vi "clear_and_initialize_fifos.vi"   [LabVIEW 2015]
uses:
  <vilib>/rvi/Emulation/niFpgaGetClockAttributes.vi
  <vilib>/rvi/Emulation/niFpgaSctlEmulationGetInTimedLoop.vi
  <vilib>/rvi/Emulation/niFpgaEmulationReportErrorSimple.vi
  <vilib>/rvi/Emulation/niFpgaEmulationIsFPGAContextNoSignature.vi
  <vilib>/rvi/FIFO/Fifo_Resource/nirvififoEmulationSetSize.vi
  <vilib>/rvi/DataTransferAndStorage/Container/Common/niFpgaContainerGetUniqueNameForEmu.vi
  <vilib>/rvi/FIFO/Fifo_Resource/nirviFifoEmulationQueueMgr.vi
  <instcachedir>/0/nirviFifoEmulationQueueMgr_E5CAEC123FF24DC58D834DCA3CDAA9B5.lvgen/nirviFifoEmulationQueueMgr_E5CAEC123FF24DC58D834DCA3CDAA9B5_002.vi
  <vilib>/rvi/Emulation/niFpgaProcessEmulError.vi
  <vilib>/rvi/DataTransferAndStorage/Container/Common/niFpgaContainerExecOnDevCompGetState.vi
  <vilib>/rvi/errors/niFpgaSetErrorForExecOnDevCompSimple.vi
  <vilib>/rvi/eio/common/nirviEmuReportErrorAndStop.vi
  <vilib>/rvi/FIFO/Fifo_Resource/nirvififoEmulationDetermineInputValidOut.vi
  <vilib>/rvi/FIFO/Fifo_Resource/nirvififoEmulationCreateLock.vi
  <vilib>/rvi/FIFO/Fifo_Resource/nirvififoEmulationObtainLock.vi
  <vilib>/rvi/FIFO/Fifo_Resource/nirvififoEmulationReleaseLock.vi
  <vilib>/rvi/occurrence/nirviWaitOnOccurrenceBase.vi
  <vilib>/rvi/errors/nirviReportUnexpectedCaseInternalError.vi
  <vilib>/rvi/errors/nirviReportUnexpectedCaseInternalError (U32).vi
  <vilib>/Utility/error.llb/Clear Errors.vi
  <vilib>/rvi/interface/RandomDataEmulation/niFpgaRandomDataHandleErrors.vi
  <vilib>/rvi/Emulation/niFpgaCriticalErrorInLSC.vi
  <instcachedir>/0/nirviFifoEmulationQueueMgr_E5CAEC123FF24DC58D834DCA3CDAA9B5.lvgen/nirviFifoEmulationQueueMgr_E5CAEC123FF24DC58D834DCA3CDAA9B5_001.vi
  <instcachedir>/0/nirviFifoEmulationQueueMgr_E5CAEC123FF24DC58D834DCA3CDAA9B5.lvgen/nirviFifoEmulationQueueMgr_E5CAEC123FF24DC58D834DCA3CDAA9B5_003.vi
  <vilib>/rvi/DataTransferAndStorage/Container/XNode/niFpgaContainer.xnode
  <vilib>/rvi/FIFO/Fifo_Resource/nirvififoEmulationClear.vi
  <vilib>/rvi/FIFO/Fifo_Resource/niFpgaFifoEmulationRefIn.vi
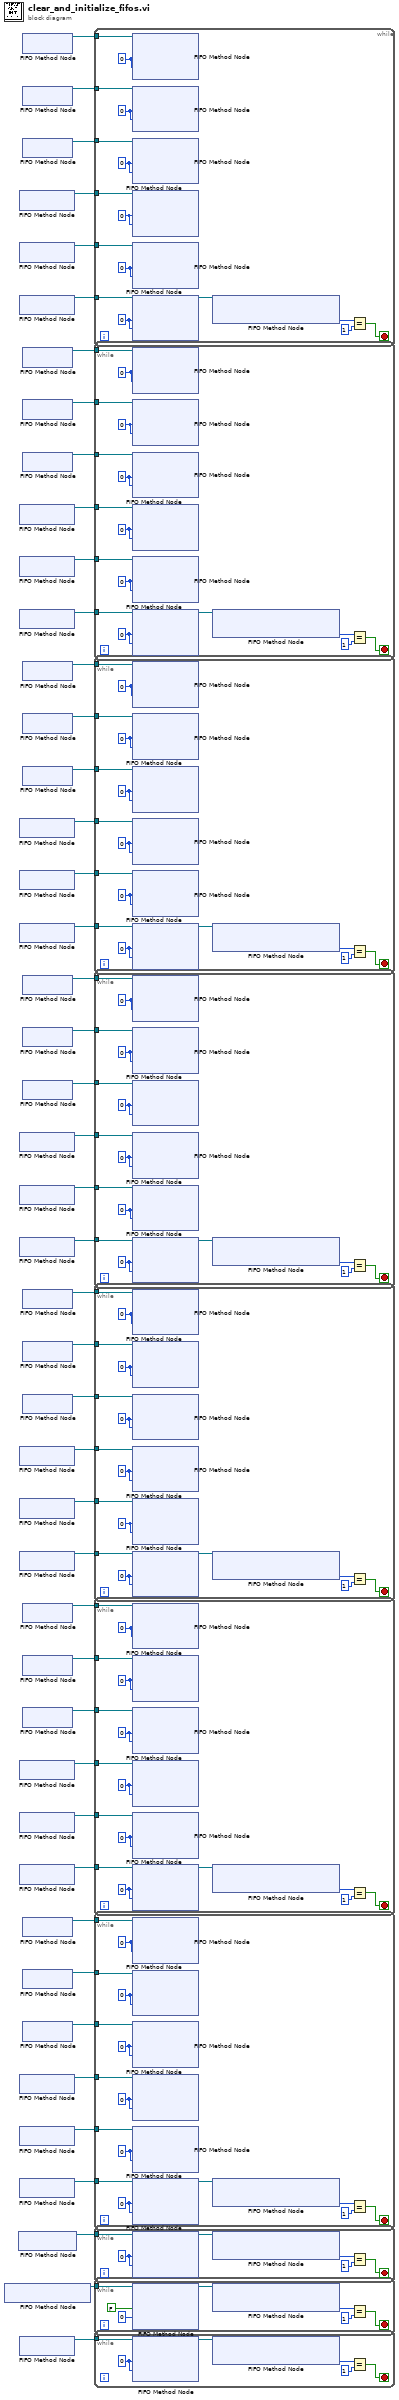
[diagram p0: block diagram]
diagram:
  n1 = xnode ("FIFO Method Node")() -> ("FIFO Out"=w2:refnum<k21>)  [unwired: 1 in]
  n2 = xnode ("FIFO Method Node")() -> ("FIFO Out"=w3:refnum<k21>)  [unwired: 1 in]
  n3 = xnode ("FIFO Method Node")() -> ("FIFO Out"=w42:refnum<k21>)  [unwired: 1 in]
  n4 = xnode ("FIFO Method Node")() -> ("FIFO Out"=w41:refnum<k21>)  [unwired: 1 in]
  n5 = xnode ("FIFO Method Node")() -> ("FIFO Out"=w40:refnum<k21>)  [unwired: 1 in]
  n6 = xnode ("FIFO Method Node")() -> ("FIFO Out"=w36:refnum<k21>)  [unwired: 1 in]
  n7 = xnode ("FIFO Method Node")() -> ("FIFO Out"=w35:refnum<k21>)  [unwired: 1 in]
  n8 = xnode ("FIFO Method Node")() -> ("FIFO Out"=w34:refnum<k21>)  [unwired: 1 in]
  n9 = xnode ("FIFO Method Node")() -> ("FIFO Out"=w30:refnum<k21>)  [unwired: 1 in]
  n10 = xnode ("FIFO Method Node")() -> ("FIFO Out"=w29:refnum<k21>)  [unwired: 1 in]
  n11 = xnode ("FIFO Method Node")() -> ("FIFO Out"=w28:refnum<k21>)  [unwired: 1 in]
  n12 = xnode ("FIFO Method Node")() -> ("FIFO Out"=w24:refnum<k21>)  [unwired: 1 in]
  n13 = xnode ("FIFO Method Node")() -> ("FIFO Out"=w23:refnum<k21>)  [unwired: 1 in]
  n14 = xnode ("FIFO Method Node")() -> ("FIFO Out"=w22:refnum<k21>)  [unwired: 1 in]
  n15 = xnode ("FIFO Method Node")() -> ("FIFO Out"=w18:refnum<k21>)  [unwired: 1 in]
  n16 = xnode ("FIFO Method Node")() -> ("FIFO Out"=w17:refnum<k21>)  [unwired: 1 in]
  n17 = xnode ("FIFO Method Node")() -> ("FIFO Out"=w16:refnum<k21>)  [unwired: 1 in]
  n18 = xnode ("FIFO Method Node")() -> ("FIFO Out"=w12:refnum<k21>)  [unwired: 1 in]
  n19 = xnode ("FIFO Method Node")() -> ("FIFO Out"=w11:refnum<k21>)  [unwired: 1 in]
  n20 = xnode ("FIFO Method Node")() -> ("FIFO Out"=w10:refnum<k21>)  [unwired: 1 in]
  n21 = xnode ("FIFO Method Node")() -> ("FIFO Out"=w6:refnum<k21>)  [unwired: 1 in]
  n22 = xnode ("FIFO Method Node")() -> ("FIFO Out"=w5:refnum<k21>)  [unwired: 1 in]
  n23 = xnode ("FIFO Method Node")() -> ("FIFO Out"=w4:refnum<k21>)  [unwired: 1 in]
  n24 = xnode ("FIFO Method Node")() -> ("FIFO Out"=w1:refnum<k21>)  [unwired: 1 in]
  n25 = xnode ("FIFO Method Node")() -> ("FIFO Out"=w45:refnum<k21>)  [unwired: 1 in]
  n26 = xnode ("FIFO Method Node")() -> ("FIFO Out"=w44:refnum<k21>)  [unwired: 1 in]
  n27 = xnode ("FIFO Method Node")() -> ("FIFO Out"=w43:refnum<k21>)  [unwired: 1 in]
  n28 = xnode ("FIFO Method Node")() -> ("FIFO Out"=w39:refnum<k21>)  [unwired: 1 in]
  n29 = xnode ("FIFO Method Node")() -> ("FIFO Out"=w38:refnum<k21>)  [unwired: 1 in]
  n30 = xnode ("FIFO Method Node")() -> ("FIFO Out"=w37:refnum<k21>)  [unwired: 1 in]
  n31 = xnode ("FIFO Method Node")() -> ("FIFO Out"=w33:refnum<k21>)  [unwired: 1 in]
  n32 = xnode ("FIFO Method Node")() -> ("FIFO Out"=w32:refnum<k21>)  [unwired: 1 in]
  n33 = xnode ("FIFO Method Node")() -> ("FIFO Out"=w31:refnum<k21>)  [unwired: 1 in]
  n34 = xnode ("FIFO Method Node")() -> ("FIFO Out"=w27:refnum<k21>)  [unwired: 1 in]
  n35 = xnode ("FIFO Method Node")() -> ("FIFO Out"=w26:refnum<k21>)  [unwired: 1 in]
  n36 = xnode ("FIFO Method Node")() -> ("FIFO Out"=w25:refnum<k21>)  [unwired: 1 in]
  n37 = xnode ("FIFO Method Node")() -> ("FIFO Out"=w21:refnum<k21>)  [unwired: 1 in]
  n38 = xnode ("FIFO Method Node")() -> ("FIFO Out"=w20:refnum<k21>)  [unwired: 1 in]
  n39 = xnode ("FIFO Method Node")() -> ("FIFO Out"=w19:refnum<k21>)  [unwired: 1 in]
  n40 = xnode ("FIFO Method Node")() -> ("FIFO Out"=w15:refnum<k21>)  [unwired: 1 in]
  n41 = xnode ("FIFO Method Node")() -> ("FIFO Out"=w14:refnum<k21>)  [unwired: 1 in]
  n42 = xnode ("FIFO Method Node")() -> ("FIFO Out"=w13:refnum<k21>)  [unwired: 1 in]
  n43 = xnode ("FIFO Method Node")() -> ("FIFO Out"=w9:refnum<k21>)  [unwired: 1 in]
  n44 = xnode ("FIFO Method Node")() -> ("FIFO Out"=w8:refnum<k21>)  [unwired: 1 in]
  n45 = xnode ("FIFO Method Node")() -> ("FIFO Out"=w7:refnum<k21>)  [unwired: 1 in]
  n46 = while {
    tunnel: w45 -> [w56]
    tunnel: w44 -> [w57]
    tunnel: w43 -> [w58]
    tunnel: w42 -> [w59]
    tunnel: w41 -> [w60]
    tunnel: w40 -> [w61]
    stop <- w47 stop-if-true
    w50 = i16 0 ("Element")
    w51 = i16 0 ("Element")
    w52 = i16 0 ("Element")
    w53 = i16 0 ("Element")
    w54 = i16 0 ("Element")
    w55 = i16 0 ("Element")
    n47 = xnode ("FIFO Method Node")("Element"=w55, "Timeout"=w55, "FIFO In"=w56) -> ()  [unwired: 2 out]
    n48 = xnode ("FIFO Method Node")("Element"=w54, "Timeout"=w54, "FIFO In"=w57) -> ()  [unwired: 2 out]
    n49 = xnode ("FIFO Method Node")("Element"=w53, "Timeout"=w53, "FIFO In"=w58) -> ()  [unwired: 2 out]
    n50 = xnode ("FIFO Method Node")("Element"=w52, "Timeout"=w52, "FIFO In"=w59) -> ()  [unwired: 2 out]
    n51 = xnode ("FIFO Method Node")("Element"=w51, "Timeout"=w51, "FIFO In"=w60) -> ()  [unwired: 2 out]
    n52 = xnode ("FIFO Method Node")("Element"=w50, "Timeout"=w50, "FIFO In"=w61) -> ("FIFO Out"=w46:refnum<k21>)  [unwired: 1 out]
    n53 = xnode ("FIFO Method Node")("FIFO In"=w46) -> ("Number of Elements to Write"=w49:u32)  [unwired: 1 out]
    n54 = Equal?(x=w49, y=u32 1 ("Number of Elements to Write")) -> (x = y?=w47:bool)
  }
  n55 = while {
    tunnel: w39 -> [w72]
    tunnel: w38 -> [w73]
    tunnel: w37 -> [w74]
    tunnel: w36 -> [w75]
    tunnel: w35 -> [w76]
    tunnel: w34 -> [w77]
    stop <- w62 stop-if-true
    w66 = i16 0 ("Element")
    w67 = i16 0 ("Element")
    w68 = i16 0 ("Element")
    w69 = i16 0 ("Element")
    w70 = i16 0 ("Element")
    w71 = i16 0 ("Element")
    n56 = xnode ("FIFO Method Node")("Element"=w71, "Timeout"=w71, "FIFO In"=w72) -> ()  [unwired: 2 out]
    n57 = xnode ("FIFO Method Node")("Element"=w70, "Timeout"=w70, "FIFO In"=w73) -> ()  [unwired: 2 out]
    n58 = xnode ("FIFO Method Node")("Element"=w69, "Timeout"=w69, "FIFO In"=w74) -> ()  [unwired: 2 out]
    n59 = xnode ("FIFO Method Node")("Element"=w68, "Timeout"=w68, "FIFO In"=w75) -> ()  [unwired: 2 out]
    n60 = xnode ("FIFO Method Node")("Element"=w67, "Timeout"=w67, "FIFO In"=w76) -> ()  [unwired: 2 out]
    n61 = xnode ("FIFO Method Node")("Element"=w66, "Timeout"=w66, "FIFO In"=w77) -> ("FIFO Out"=w65:refnum<k21>)  [unwired: 1 out]
    n62 = xnode ("FIFO Method Node")("FIFO In"=w65) -> ("Number of Elements to Write"=w64:u32)  [unwired: 1 out]
    n63 = Equal?(x=w64, y=u32 1 ("Number of Elements to Write")) -> (x = y?=w62:bool)
  }
  n64 = while {
    tunnel: w33 -> [w88]
    tunnel: w32 -> [w89]
    tunnel: w31 -> [w90]
    tunnel: w30 -> [w91]
    tunnel: w29 -> [w92]
    tunnel: w28 -> [w93]
    stop <- w78 stop-if-true
    w82 = i16 0 ("Element")
    w83 = i16 0 ("Element")
    w84 = i16 0 ("Element")
    w85 = i16 0 ("Element")
    w86 = i16 0 ("Element")
    w87 = i16 0 ("Element")
    n65 = xnode ("FIFO Method Node")("Element"=w87, "Timeout"=w87, "FIFO In"=w88) -> ()  [unwired: 2 out]
    n66 = xnode ("FIFO Method Node")("Element"=w86, "Timeout"=w86, "FIFO In"=w89) -> ()  [unwired: 2 out]
    n67 = xnode ("FIFO Method Node")("Element"=w85, "Timeout"=w85, "FIFO In"=w90) -> ()  [unwired: 2 out]
    n68 = xnode ("FIFO Method Node")("Element"=w84, "Timeout"=w84, "FIFO In"=w91) -> ()  [unwired: 2 out]
    n69 = xnode ("FIFO Method Node")("Element"=w83, "Timeout"=w83, "FIFO In"=w92) -> ()  [unwired: 2 out]
    n70 = xnode ("FIFO Method Node")("Element"=w82, "Timeout"=w82, "FIFO In"=w93) -> ("FIFO Out"=w81:refnum<k21>)  [unwired: 1 out]
    n71 = xnode ("FIFO Method Node")("FIFO In"=w81) -> ("Number of Elements to Write"=w80:u32)  [unwired: 1 out]
    n72 = Equal?(x=w80, y=u32 1 ("Number of Elements to Write")) -> (x = y?=w78:bool)
  }
  n73 = while {
    tunnel: w27 -> [w104]
    tunnel: w26 -> [w105]
    tunnel: w25 -> [w106]
    tunnel: w24 -> [w107]
    tunnel: w23 -> [w108]
    tunnel: w22 -> [w109]
    stop <- w94 stop-if-true
    w98 = i16 0 ("Element")
    w99 = i16 0 ("Element")
    w100 = i16 0 ("Element")
    w101 = i16 0 ("Element")
    w102 = i16 0 ("Element")
    w103 = i16 0 ("Element")
    n74 = xnode ("FIFO Method Node")("Element"=w103, "Timeout"=w103, "FIFO In"=w104) -> ()  [unwired: 2 out]
    n75 = xnode ("FIFO Method Node")("Element"=w102, "Timeout"=w102, "FIFO In"=w105) -> ()  [unwired: 2 out]
    n76 = xnode ("FIFO Method Node")("Element"=w101, "Timeout"=w101, "FIFO In"=w106) -> ()  [unwired: 2 out]
    n77 = xnode ("FIFO Method Node")("Element"=w100, "Timeout"=w100, "FIFO In"=w107) -> ()  [unwired: 2 out]
    n78 = xnode ("FIFO Method Node")("Element"=w99, "Timeout"=w99, "FIFO In"=w108) -> ()  [unwired: 2 out]
    n79 = xnode ("FIFO Method Node")("Element"=w98, "Timeout"=w98, "FIFO In"=w109) -> ("FIFO Out"=w97:refnum<k21>)  [unwired: 1 out]
    n80 = xnode ("FIFO Method Node")("FIFO In"=w97) -> ("Number of Elements to Write"=w96:u32)  [unwired: 1 out]
    n81 = Equal?(x=w96, y=u32 1 ("Number of Elements to Write")) -> (x = y?=w94:bool)
  }
  n82 = while {
    tunnel: w21 -> [w120]
    tunnel: w20 -> [w121]
    tunnel: w19 -> [w122]
    tunnel: w18 -> [w123]
    tunnel: w17 -> [w124]
    tunnel: w16 -> [w125]
    stop <- w110 stop-if-true
    w114 = i16 0 ("Element")
    w115 = i16 0 ("Element")
    w116 = i16 0 ("Element")
    w117 = i16 0 ("Element")
    w118 = i16 0 ("Element")
    w119 = i16 0 ("Element")
    n83 = xnode ("FIFO Method Node")("Element"=w119, "Timeout"=w119, "FIFO In"=w120) -> ()  [unwired: 2 out]
    n84 = xnode ("FIFO Method Node")("Element"=w118, "Timeout"=w118, "FIFO In"=w121) -> ()  [unwired: 2 out]
    n85 = xnode ("FIFO Method Node")("Element"=w117, "Timeout"=w117, "FIFO In"=w122) -> ()  [unwired: 2 out]
    n86 = xnode ("FIFO Method Node")("Element"=w116, "Timeout"=w116, "FIFO In"=w123) -> ()  [unwired: 2 out]
    n87 = xnode ("FIFO Method Node")("Element"=w115, "Timeout"=w115, "FIFO In"=w124) -> ()  [unwired: 2 out]
    n88 = xnode ("FIFO Method Node")("Element"=w114, "Timeout"=w114, "FIFO In"=w125) -> ("FIFO Out"=w113:refnum<k21>)  [unwired: 1 out]
    n89 = xnode ("FIFO Method Node")("FIFO In"=w113) -> ("Number of Elements to Write"=w112:u32)  [unwired: 1 out]
    n90 = Equal?(x=w112, y=u32 1 ("Number of Elements to Write")) -> (x = y?=w110:bool)
  }
  n91 = while {
    tunnel: w15 -> [w136]
    tunnel: w14 -> [w137]
    tunnel: w13 -> [w138]
    tunnel: w12 -> [w139]
    tunnel: w11 -> [w140]
    tunnel: w10 -> [w141]
    stop <- w126 stop-if-true
    w130 = i16 0 ("Element")
    w131 = i16 0 ("Element")
    w132 = i16 0 ("Element")
    w133 = i16 0 ("Element")
    w134 = i16 0 ("Element")
    w135 = i16 0 ("Element")
    n92 = xnode ("FIFO Method Node")("Element"=w135, "Timeout"=w135, "FIFO In"=w136) -> ()  [unwired: 2 out]
    n93 = xnode ("FIFO Method Node")("Element"=w134, "Timeout"=w134, "FIFO In"=w137) -> ()  [unwired: 2 out]
    n94 = xnode ("FIFO Method Node")("Element"=w133, "Timeout"=w133, "FIFO In"=w138) -> ()  [unwired: 2 out]
    n95 = xnode ("FIFO Method Node")("Element"=w132, "Timeout"=w132, "FIFO In"=w139) -> ()  [unwired: 2 out]
    n96 = xnode ("FIFO Method Node")("Element"=w131, "Timeout"=w131, "FIFO In"=w140) -> ()  [unwired: 2 out]
    n97 = xnode ("FIFO Method Node")("Element"=w130, "Timeout"=w130, "FIFO In"=w141) -> ("FIFO Out"=w129:refnum<k21>)  [unwired: 1 out]
    n98 = xnode ("FIFO Method Node")("FIFO In"=w129) -> ("Number of Elements to Write"=w128:u32)  [unwired: 1 out]
    n99 = Equal?(x=w128, y=u32 1 ("Number of Elements to Write")) -> (x = y?=w126:bool)
  }
  n100 = while {
    tunnel: w9 -> [w152]
    tunnel: w8 -> [w153]
    tunnel: w7 -> [w154]
    tunnel: w6 -> [w155]
    tunnel: w5 -> [w156]
    tunnel: w4 -> [w157]
    stop <- w142 stop-if-true
    w146 = i16 0 ("Element")
    w147 = i16 0 ("Element")
    w148 = i16 0 ("Element")
    w149 = i16 0 ("Element")
    w150 = i16 0 ("Element")
    w151 = i16 0 ("Element")
    n101 = xnode ("FIFO Method Node")("Element"=w151, "Timeout"=w151, "FIFO In"=w152) -> ()  [unwired: 2 out]
    n102 = xnode ("FIFO Method Node")("Element"=w150, "Timeout"=w150, "FIFO In"=w153) -> ()  [unwired: 2 out]
    n103 = xnode ("FIFO Method Node")("Element"=w149, "Timeout"=w149, "FIFO In"=w154) -> ()  [unwired: 2 out]
    n104 = xnode ("FIFO Method Node")("Element"=w148, "Timeout"=w148, "FIFO In"=w155) -> ()  [unwired: 2 out]
    n105 = xnode ("FIFO Method Node")("Element"=w147, "Timeout"=w147, "FIFO In"=w156) -> ()  [unwired: 2 out]
    n106 = xnode ("FIFO Method Node")("Element"=w146, "Timeout"=w146, "FIFO In"=w157) -> ("FIFO Out"=w145:refnum<k21>)  [unwired: 1 out]
    n107 = xnode ("FIFO Method Node")("FIFO In"=w145) -> ("Number of Elements to Write"=w144:u32)  [unwired: 1 out]
    n108 = Equal?(x=w144, y=u32 1 ("Number of Elements to Write")) -> (x = y?=w142:bool)
  }
  n109 = while {
    tunnel: w3 -> [w163]
    stop <- w158 stop-if-true
    w162 = i16 0 ("Element")
    n110 = xnode ("FIFO Method Node")("Element"=w162, "Timeout"=w162, "FIFO In"=w163) -> ("FIFO Out"=w161:refnum<k21>)  [unwired: 1 out]
    n111 = xnode ("FIFO Method Node")("FIFO In"=w161) -> ("Number of Elements to Write"=w160:u32)  [unwired: 1 out]
    n112 = Equal?(x=w160, y=u32 1 ("Number of Elements to Write")) -> (x = y?=w158:bool)
  }
  n113 = while {
    tunnel: w2 -> [w170]
    stop <- w165 stop-if-true
    n114 = xnode ("FIFO Method Node")("Element"=FALSE, "Timeout"=i16 0 ("Element"), "FIFO In"=w170) -> ("FIFO Out"=w168:refnum<k21>)  [unwired: 1 out]
    n115 = xnode ("FIFO Method Node")("FIFO In"=w168) -> ("Number of Elements to Write"=w167:u32)  [unwired: 1 out]
    n116 = Equal?(x=w167, y=u32 1 ("Number of Elements to Write")) -> (x = y?=w165:bool)
  }
  n117 = while {
    tunnel: w1 -> [w176]
    stop <- w171 stop-if-true
    w175 = i16 0 ("Element")
    n118 = xnode ("FIFO Method Node")("Element"=w175, "Timeout"=w175, "FIFO In"=w176) -> ("FIFO Out"=w174:refnum<k21>)  [unwired: 1 out]
    n119 = xnode ("FIFO Method Node")("FIFO In"=w174) -> ("Number of Elements to Write"=w173:u32)  [unwired: 1 out]
    n120 = Equal?(x=w173, y=u32 1 ("Number of Elements to Write")) -> (x = y?=w171:bool)
  }
